vi "Save DAC Configuration.vi"(8 "error in":errorcluster, 10 "Config File refnum in":T1, 11 "DAC DC Supply in":refnum<class "DAC DC Supply.lvclass">) -> (0 "error out":errorcluster, 2 "Config File refnum out":T1, 3 "DAC DC Supply out":refnum<class "DAC DC Supply.lvclass">)   [LabVIEW 2019, in "DAC.lvlib" / "DAC DC Supply.lvclass"]
uses:
  DAC DC Supply.lvclass
  C:/Users/krio/Documents/LV_Projects/test-stand/App/DAC/DAC.lvclass
  <vilib>/Utility/config.llb/Config Data RefNum.ctl
  DAC.lvclass/DAC.ctl
  DAC DC Supply.lvclass/DAC DC Supply.ctl
  <vilib>/Utility/config.llb/Write Key (String).vi
  DAC.lvclass
  <vilib>/Utility/config.llb/NI_LVConfig.lvlib
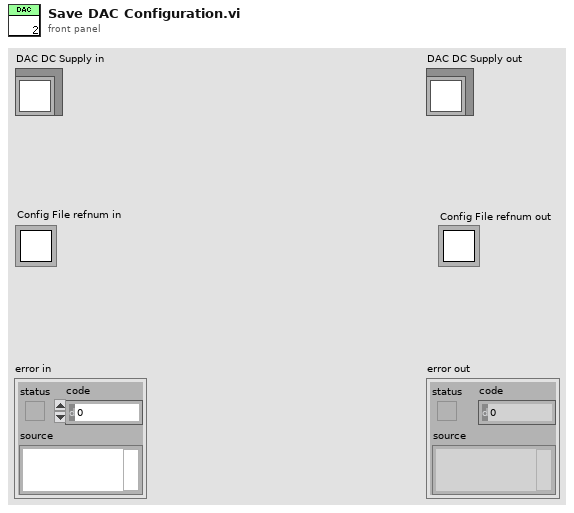
[diagram p1: front panel]
types:
  T1 = typedef "NI_LVConfig.lvlib/Config Data RefNum.ctl" = refnum<k1>
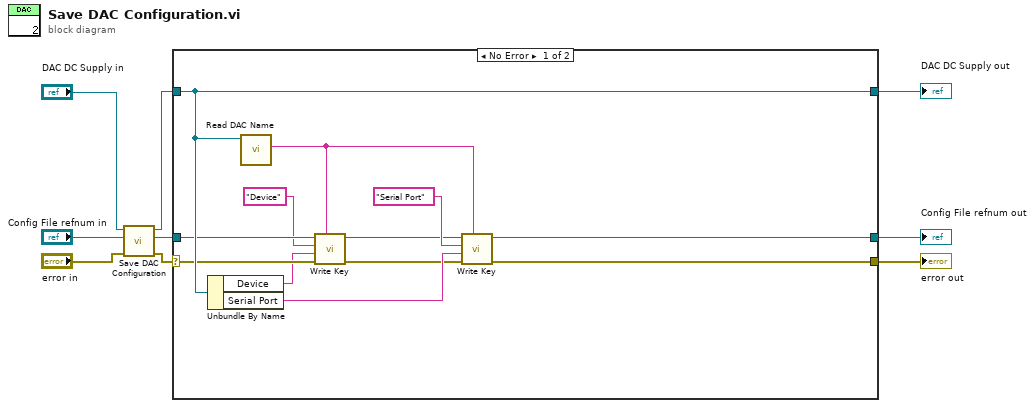
[diagram p0: block diagram]
diagram:
  n1 = call-parent "Save DAC Configuration.vi"("error in"="error in", "Config File refnum in"="Config File refnum in", "DAC in"="DAC DC Supply in") -> ("error out"=w4:errorcluster, "Config File refnum out"=w5:T1, "DAC out"=w6:refnum<class "DAC DC Supply.lvclass">)  [unwired: 6 in]
  n2 = case shown="No Error" w4 {
    selector: w4 -> [w17 w24]
    tunnel: [w10 w24] -> w1
    tunnel: [w21 w23] -> w3
    tunnel: w6 -> [w21 w23]
    tunnel: w5 -> [w18 w22]
    tunnel: [w11 w22] -> w2
    frame No Error {
      n3 = Unbundle By Name(w21) -> ("Device"=w13:string, "Serial Port"=w19:string)
      n4 = call "Read DAC Name.vi"("DAC in"=w21) -> ("DAC Name"=w12:string)  [unwired: 8 in, 2 out]
      n5 = call-poly <vilib>:"Write Key.vi"("section"=w12, "error in (no error)"=w17, "value"=w13, "key"="Device", "refnum"=w18) -> ("error out"=w15:errorcluster, "refnum out"=w16:T1)  [unwired: 4 in, 1 out]
      n6 = call-poly <vilib>:"Write Key.vi"("section"=w12, "error in (no error)"=w15, "value"=w19, "key"="Serial Port", "refnum"=w16) -> ("error out"=w10:errorcluster, "refnum out"=w11:T1)  [unwired: 4 in, 1 out]
    }
    frame Error {
    }
  }
  "error out" <- w1
  "DAC DC Supply out" <- w3
  "Config File refnum out" <- w2
